vi "Skip Fire Settings Write.vi"(8 "error in":errorcluster, 9 "Device Inputs":dbl[](array[numeric]), 10 "DCM Ref":refnum<class "DCM - RT.lvclass">, 11 "Skip Fire":T1={"Skip Fire Enabled"=FALSE, "FIFO Indexes"={"Write"={"Setup"=[{"Enable"=-1, "Total Cycles"=-1, "On Cycles"=-1, "TDC Offset [CAD]"=-1}, {"Enable"=-1, "Total Cycles"=-1, "On Cycles"=-1, "TDC Offset [CAD]"=-1}, {"Enable"=-1, "Total Cycles"=-1, "On Cycles"=-1, "TDC Offset [CAD]"=-1}, {"Enable"=-1, "Total Cycles"=-1, "On Cycles"=-1, "TDC Offset [CAD]"=-1}, {"Enable"=-1, "Total Cycles"=-1, "On Cycles"=-1, "TDC Offset [CAD]"=-1}, {"Enable"=-1, "Total Cycles"=-1, "On Cycles"=-1, "TDC Offset [CAD]"=-1}, {"Enable"=-1, "Total Cycles"=-1, "On Cycles"=-1, "TDC Offset [CAD]"=-1}, {"Enable"=-1, "Total Cycles"=-1, "On Cycles"=-1, "TDC Offset [CAD]"=-1}]}}}) -> (0 "error out":errorcluster)   [LabVIEW 2016, in "DCM Engine.lvlib"]
uses:
  DCM Engine.lvlib
  Built/DCM Classes Packed/Pharlap/C/DCM-Classes.lvlibp/DCM/Rev0/RT/DCM - RT.lvclass
  Shared/Types/Skip Fire.ctl
  Shared/Types/Skip Fire Setup Indexes.ctl
  Built/DCM Classes Packed/Pharlap/C/DCM-Classes.lvlibp/DCM/Skip Fire/RT/DCM - RT - Skip Fire.lvlib
  DCM Shared.lvlib
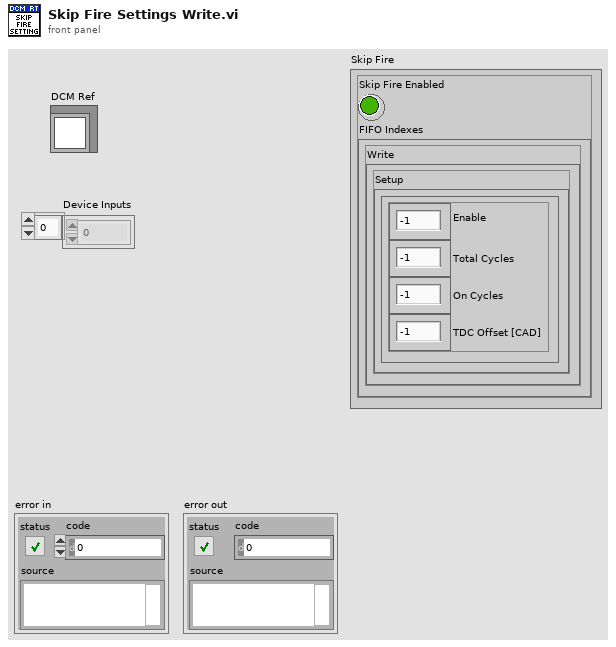
[diagram p1: front panel]
types:
  T1 = typedef "DCM Shared.lvlib/Skip Fire.ctl" = cluster{"Skip Fire Enabled":bool, "FIFO Indexes":cluster{"Write":cluster{"Setup":T2[]}}}
  T2 = typedef "DCM Shared.lvlib/Skip Fire Setup Indexes.ctl" = cluster{"Enable":i32, "Total Cycles":i32, "On Cycles":i32, "TDC Offset [CAD]":i32}
  T3 = typedef "DCM-Classes.lvlibp/DCM - RT - Skip Fire.lvlib/Skip Fire Setup.ctl" = cluster{"Enable":bool, "Total Cycles":u8, "On Cycles":u8, "TDC Offset [CAD]":sgl}
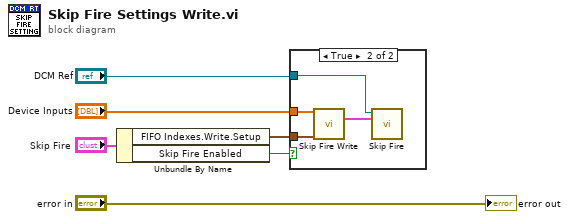
[diagram p0: block diagram]
diagram:
  n1 = Unbundle By Name("Skip Fire") -> ("FIFO Indexes.Write.Setup"=w2:T2[], "Skip Fire Enabled"=w1:bool)
  n2 = case shown="True" w1 {
    tunnel: "Device Inputs" -> [_ w10]
    tunnel: "DCM Ref" -> [_ w7]
    tunnel: w2 -> [_ w8]
    frame False {
    }
    frame True {
      n3 = call "Skip Fire Write.vi"("Device Inputs"=w10, "Setup Indexes"=w8) -> ("Setup"=w9:T3[])  [unwired: 13 in]
      n4 = call "Skip Fire.vi"("Skip Fire Setup"=w9, "DCM Reference"=w7) -> ()  [unwired: 10 in]
    }
  }
  "error out" <- "error in"
